vi "getCurrentF.vi"(0 "AcTension(all)":dbl[](array[numeric]), 2 "A Trunk Matrix":T1, 3 "A Pelvic Matrix":T1) -> (5 "ActF Trunk":dbl[](array[numeric]), 7 "ActF Pelvis":dbl[](array[numeric]))   [LabVIEW 2017]
uses:
  <vilib>/Analysis/Matrix/Datatypes/RealMatrix.ctl
  <vilib>/Analysis/Matrix/Numeric/Conversions/Array To Matrix - RA.vi
  <vilib>/Analysis/Matrix/Numeric/Multiply/Multiply - RM,RM.vi
  <vilib>/Analysis/Matrix/NI_Matrix.lvlib
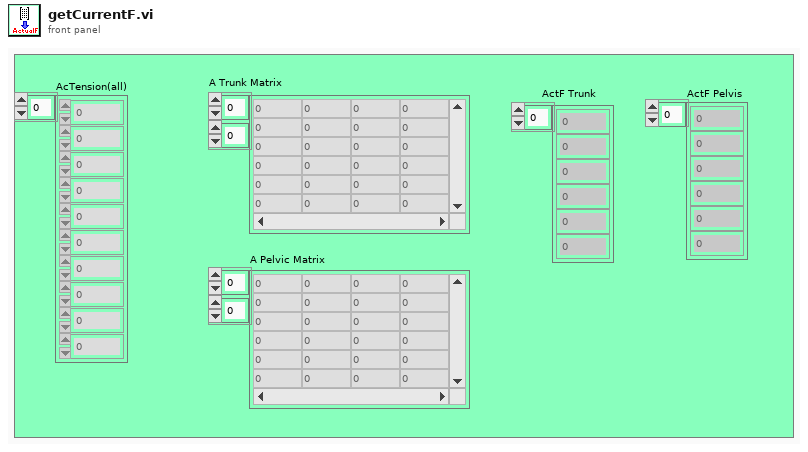
[diagram p1: front panel]
types:
  T1 = typedef "NI_Matrix.lvlib/RealMatrix.ctl" = dbl[][]
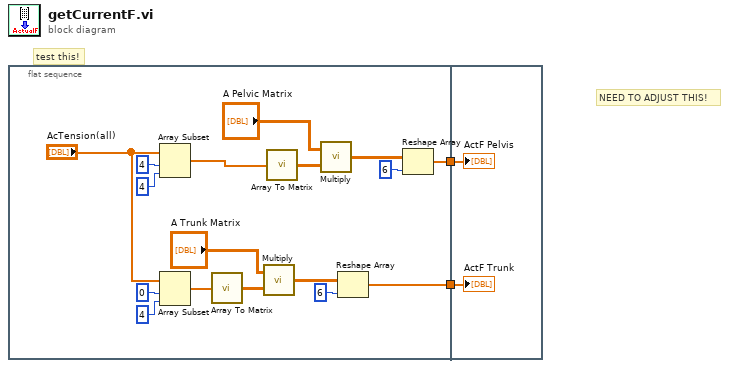
[diagram p0: block diagram]
diagram:
  # "NEED TO ADJUST THIS!"
  # "test this!"
  n1 = flat-sequence {
    tunnel: [w14] -> w2
    tunnel: [w10] -> w1
    tunnel: w2 -> [w21]
    tunnel: w1 -> [w20]
    frame #0 {
      n2 = Array Subset(array="AcTension(all)", index=4, length=4) -> (w3:dbl[])
      n3 = Array Subset(array="AcTension(all)", index=0, length=4) -> (w5:dbl[])
      n4 = call-poly <vilib>:"Array To Matrix.vi"("Real 1D Array"=w5) -> ("Real Matrix (Column Vector)"=w18:T1)
      n5 = call-poly <vilib>:"Multiply.vi"("Real Matrix B"=w18, "Real Matrix A"="A Trunk Matrix") -> ("A * B"=w15:T1)
      n6 = call-poly <vilib>:"Array To Matrix.vi"("Real 1D Array"=w3) -> ("Real Matrix (Column Vector)"=w17:T1)
      n7 = call-poly <vilib>:"Multiply.vi"("Real Matrix B"=w17, "Real Matrix A"="A Pelvic Matrix") -> ("A * B"=w12:T1)
      n8 = Reshape Array(w15, 6 ("dimension size")) -> (w14:dbl[])
      n9 = Reshape Array(w12, 6 ("dimension size")) -> (w10:dbl[])
    }
    frame #1 {
      "ActF Trunk" <- w21
      "ActF Pelvis" <- w20
    }
  }
